vi "质控参数读取.vi"(7 "section":string="氨氮质控参数", 8 "error in (no error)":errorcluster caption="错误输入（无错误）") -> (0 "error out":errorcluster caption="错误输出", 3 "参数":T1)   [LabVIEW 2016, in "质控单元.lvlib"]
uses:
  <vilib>/Utility/config.llb/Read Key (Double).vi
  <vilib>/Utility/config.llb/NI_LVConfig.lvlib
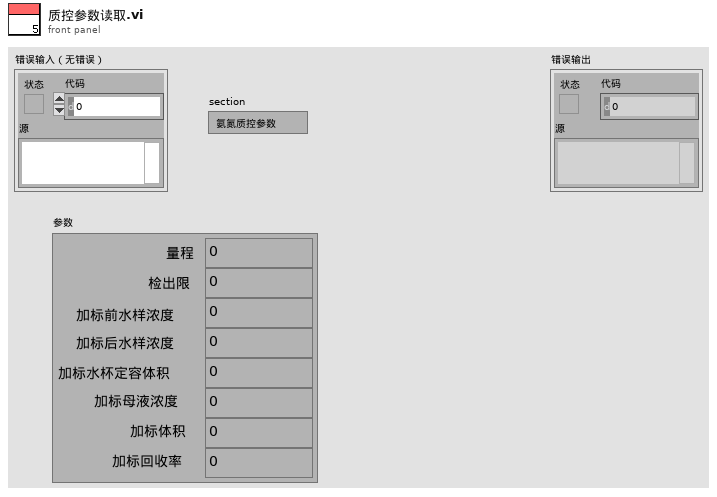
[diagram p1: front panel]
types:
  T1 = cluster{"量程":dbl, "检出限":dbl, "加标前水样浓度":dbl, "加标后水样浓度":dbl, "加标水杯定容体积":dbl, "加标母液浓度":dbl, "加标体积":dbl, "加标回收率":dbl}
  T2 = typedef "NI_LVConfig.lvlib/Config Data RefNum.ctl" = refnum<k1>
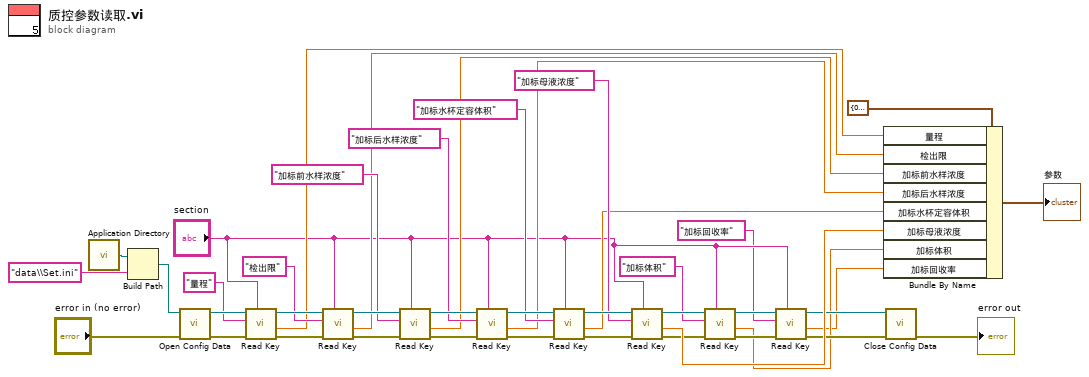
[diagram p0: block diagram]
diagram:
  n1 = call <vilib>:"Application Directory.vi"() -> ("Application Directory"=w40:path)
  n2 = Build Path(base path=w40, name or relative path="data\\Set.ini" ("名称或相对路径")) -> (appended path=w38:path)
  n3 = call <vilib>:"Open Config Data.vi"("error in (no error)"="error in (no error)", "configuration file path"=w38) -> ("error out"=w41:errorcluster, "refnum"=w42:T2)  [unwired: 7 in, 1 out]
  n4 = call-poly <vilib>:"Read Key.vi"("section"="section", "error in (no error)"=w41, "key"="量程", "refnum"=w42) -> ("error out"=w35:errorcluster, "value"=w21:dbl, "refnum out"=w36:T2)  [unwired: 4 in, 1 out]
  n5 = call-poly <vilib>:"Read Key.vi"("section"="section", "error in (no error)"=w35, "key"="检出限", "refnum"=w36) -> ("error out"=w33:errorcluster, "value"=w20:dbl, "refnum out"=w34:T2)  [unwired: 4 in, 1 out]
  n6 = call-poly <vilib>:"Read Key.vi"("section"="section", "error in (no error)"=w33, "key"="加标前水样浓度", "refnum"=w34) -> ("error out"=w27:errorcluster, "value"=w19:dbl, "refnum out"=w28:T2)  [unwired: 4 in, 1 out]
  n7 = call-poly <vilib>:"Read Key.vi"("section"="section", "error in (no error)"=w27, "key"="加标后水样浓度", "refnum"=w28) -> ("error out"=w30:errorcluster, "value"=w18:dbl, "refnum out"=w29:T2)  [unwired: 4 in, 1 out]
  n8 = call-poly <vilib>:"Read Key.vi"("section"="section", "error in (no error)"=w30, "key"="加标水杯定容体积", "refnum"=w29) -> ("error out"=w32:errorcluster, "value"=w17:dbl, "refnum out"=w31:T2)  [unwired: 4 in, 1 out]
  n9 = call-poly <vilib>:"Read Key.vi"("section"="section", "error in (no error)"=w32, "key"="加标母液浓度", "refnum"=w31) -> ("error out"=w7:errorcluster, "value"=w16:dbl, "refnum out"=w9:T2)  [unwired: 4 in, 1 out]
  n10 = call-poly <vilib>:"Read Key.vi"("section"="section", "error in (no error)"=w7, "key"="加标体积", "refnum"=w9) -> ("error out"=w6:errorcluster, "value"=w4:dbl, "refnum out"=w11:T2)  [unwired: 4 in, 1 out]
  n11 = call-poly <vilib>:"Read Key.vi"("section"="section", "error in (no error)"=w6, "key"="加标回收率", "refnum"=w11) -> ("error out"=w5:errorcluster, "value"=w3:dbl, "refnum out"=w8:T2)  [unwired: 4 in, 1 out]
  n12 = Bundle By Name(cluster=T1 {"量程"=0.0, "检出限"=0.0, "加标前水样浓度"=0.0, "加标后水样浓度"=0.0, "加标水杯定容体积"=0.0, "加标母液浓度"=0.0, "加标体积"=0.0, "加标回收率"=0.0} ("参数"), "量程"=w21, "检出限"=w20, "加标前水样浓度"=w19, "加标后水样浓度"=w18, "加标水杯定容体积"=w17, "加标母液浓度"=w16, "加标体积"=w4, "加标回收率"=w3) -> (→"参数":T1)
  n13 = call <vilib>:"Close Config Data.vi"("error in (no error)"=w5, "refnum"=w8) -> ("error out"=→"error out":errorcluster)  [unwired: 8 in, 1 out]
